vi "ManMarkZagueiro2.vi"(8 "Our Robot":T1={"id"=0, "function"=enum."Attacker", "x"=0.0, "y"=0.0, "orientation"=0.0, "v_tangent"=0.0, "v_normal"=0.0, "v_ang"=0.0, "kick_x"=0.0, "kick_z"=0.0, "dribble"=FALSE, "Timestamp"=timestamp(0 s since 1904-01-01), "estimatives"={"est_v_tangent"=0.0, "est_v_normal"=0.0, "est_vx"=0.0, "est_vy"=0.0, "Pos Robot Est"=[]}, "dest_x_kick"=0.0, "dest_y_kick"=0.0, "Gap Coord"=[], "States"=enum."GoToTangent", "Path "=[], "Path  Smooth"=[], "Dest"=[]}, 10 "IA Input":T6={"our_robots"=[], "enemy_robots"=[], "balls"=[], "geometry"={"line_width"=0, "field_length"=0, "field_width"=0, "boundary_width"=0, "referee_width"=0, "goal_width"=0, "goal_depth"=0, "goal_wall_width"=0, "center_circle_radius"=0, "defense_radius"=0, "defense_stretch"=0, "free_kick_from_defense_dist"=0, "penalty_spot_from_field_line_dist"=0, "penalty_line_from_spot_dist"=0}, "IA Judge"={"stage"="", "command"="", "our_goalie_id"=0.0, "enemy_goalie_id"=0.0, "command enum"=enum."Halt", "Time"=enum."Azul"}, "Received Timestamp"=timestamp(0 s since 1904-01-01), "Events"={"Touch"=FALSE, "Ball out"=FALSE, "id touch"=0.0, "Ball out of \nVision"=FALSE, "Ball inside \nGoalie area"=FALSE, "Robot not responding"=FALSE, "Robots responding status"=[1.0, 1.0, 1.0, 1.0, 1.0, 1.0], "Enemy Ball \nPossession"=FALSE, "Pass State"=FALSE, "id end of pass"=0.0, "Kick"=FALSE, "Id ini Possession"=0.0, "Ball Possesion"=FALSE, "Id Possesion"=0.0}}) -> (2 "Robot out":T1={"id"=0, "function"=enum."Attacker", "x"=0.0, "y"=0.0, "orientation"=0.0, "v_tangent"=0.0, "v_normal"=0.0, "v_ang"=0.0, "kick_x"=0.0, "kick_z"=0.0, "dribble"=FALSE, "Timestamp"=timestamp(0 s since 1904-01-01), "estimatives"={"est_v_tangent"=0.0, "est_v_normal"=0.0, "est_vx"=0.0, "est_vy"=0.0, "Pos Robot Est"=[]}, "dest_x_kick"=0.0, "dest_y_kick"=0.0, "Gap Coord"=[], "States"=enum."GoToTangent", "Path "=[], "Path  Smooth"=[], "Dest"=[]})   [LabVIEW 2017]
uses:
  Core/Field Size.ctl
  Core/AI Input.ctl
  Core/AI Robot.ctl
  Functions Enum.ctl
  AttackerStates.ctl
  Path Planning/RRT/PathDests.ctl
  Path Planning/RRT/PathDest.ctl
  Core/AI Ball.ctl
  Core/AI Judge.ctl
  Command Enum.ctl
  Util/Events/Events.ctl
panel:
  in  "Field Size in":T8
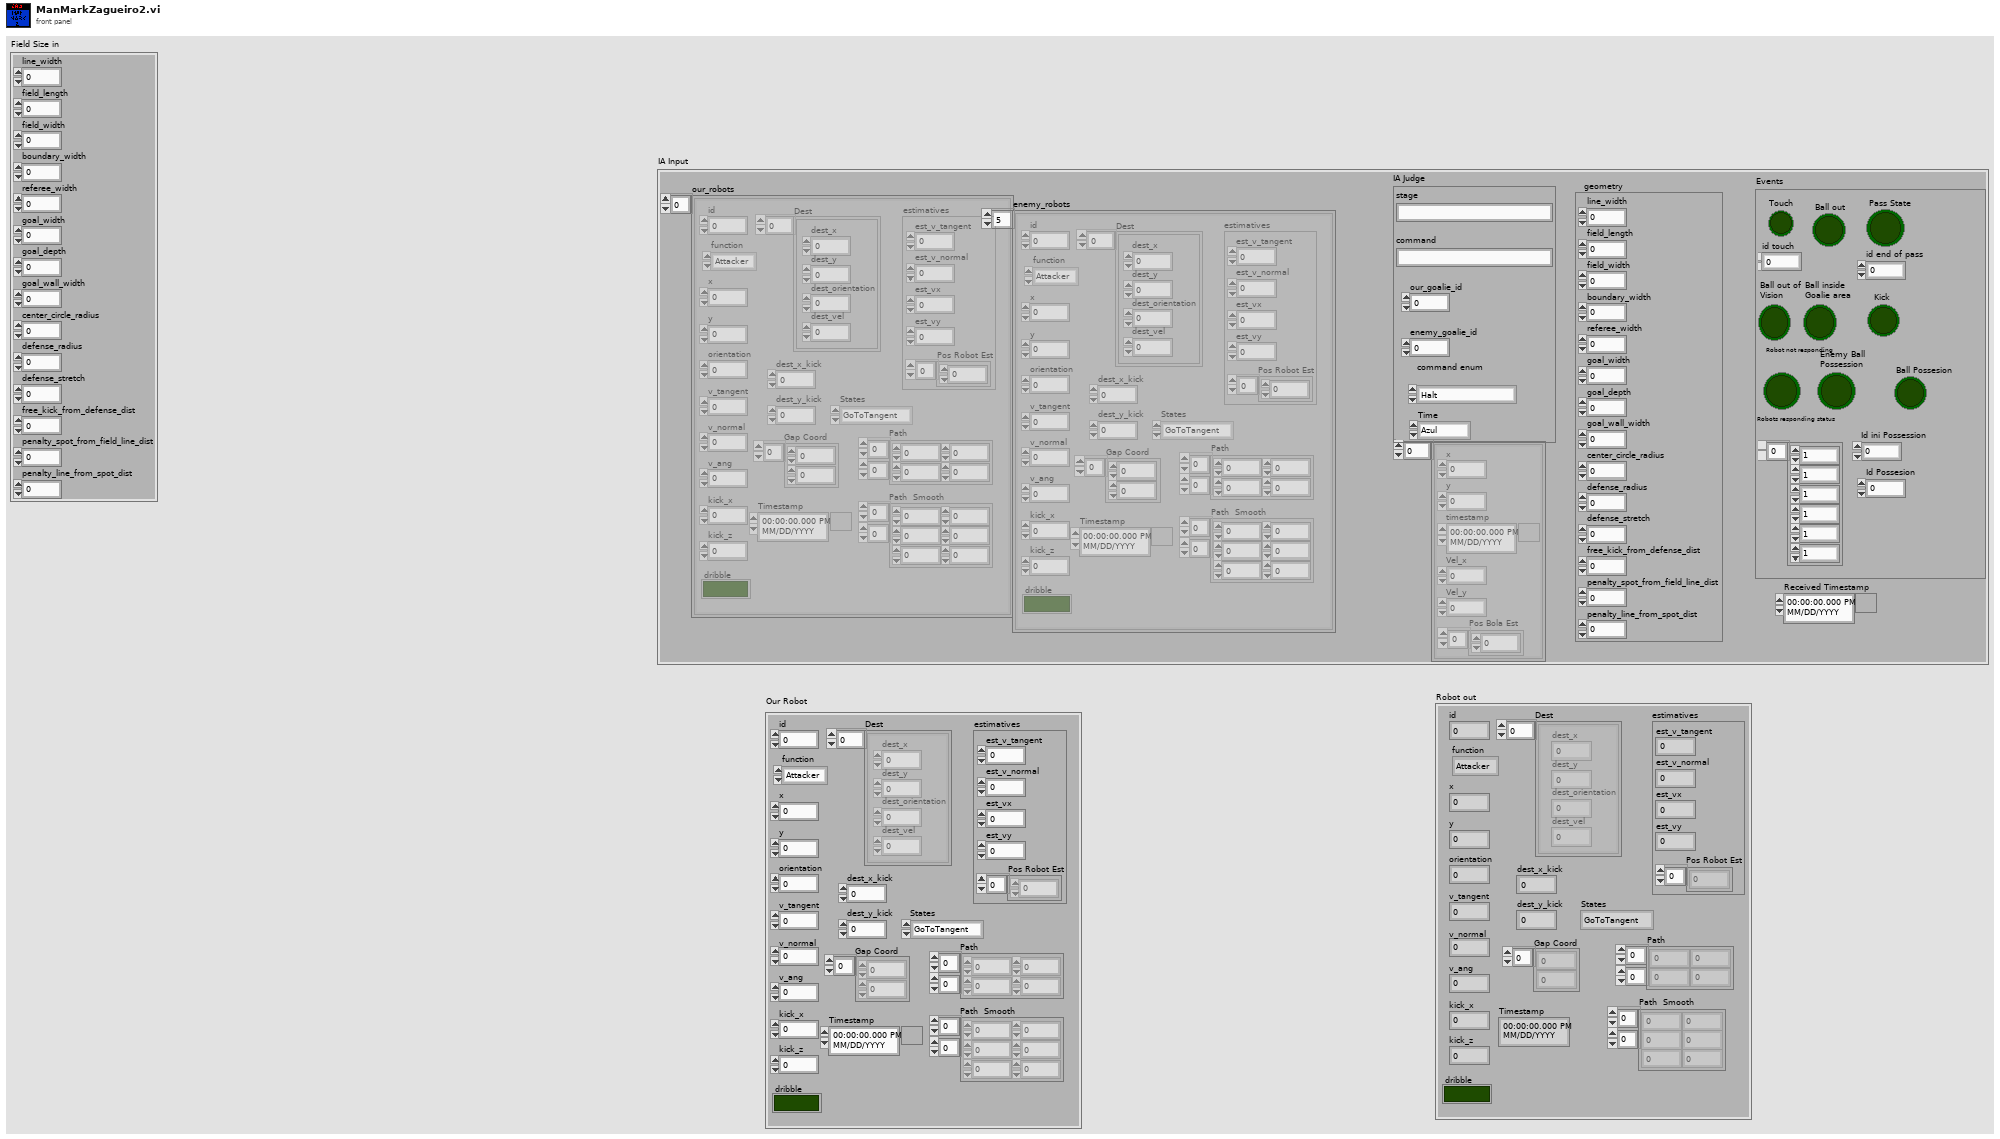
[diagram p1: front panel]
types:
  T1 = typedef "AI Robot.ctl" = cluster{"id":u32, "function":T2, "x":dbl, "y":dbl, "orientation":dbl, "v_tangent":dbl, "v_normal":dbl, "v_ang":dbl, "kick_x":dbl, "kick_z":dbl, "dribble":bool, "Timestamp":timestamp, "estimatives":cluster{"est_v_tangent":dbl, "est_v_normal":dbl, "est_vx":dbl, "est_vy":dbl, "Pos Robot Est":dbl[]}, "dest_x_kick":dbl, "dest_y_kick":dbl, "Gap Coord":dbl[], "States":T3, "Path ":dbl[][], "Path  Smooth":dbl[][], "Dest":T4}
  T2 = typedef "Functions Enum.ctl" = enum16{"Attacker", "Goalie", "Defender", "Striker", "Goto 0", "Dummy", "Kicker", "ZigZag"}
  T3 = typedef "AttackerStates.ctl" = enum16{"Pass", "GoToTangent", "BallGetting", "GoToKick", ""}
  T4 = typedef "PathDests.ctl" = T5[]
  T5 = typedef "PathDest.ctl" = cluster{"dest_x":dbl, "dest_y":dbl, "dest_orientation":dbl, "dest_vel":dbl}
  T6 = typedef "AI Input.ctl" = cluster{"our_robots":T1[], "enemy_robots":T1[], "balls":T7[], "geometry":T8, "IA Judge":T9, "Received Timestamp":timestamp, "Events":T11}
  T7 = typedef "AI Ball.ctl" = cluster{"x":dbl, "y":dbl, "timestamp":timestamp, "Vel_x":dbl, "Vel_y":dbl, "Pos Bola Est":dbl[]}
  T8 = typedef "Field Size.ctl" = cluster{"line_width":u32, "field_length":u32, "field_width":u32, "boundary_width":u32, "referee_width":u32, "goal_width":u32, "goal_depth":u32, "goal_wall_width":u32, "center_circle_radius":u32, "defense_radius":u32, "defense_stretch":u32, "free_kick_from_defense_dist":u32, "penalty_spot_from_field_line_dist":u32, "penalty_line_from_spot_dist":u32}
  T9 = typedef "AI Judge.ctl" = cluster{"stage":string, "command":string, "our_goalie_id":dbl, "enemy_goalie_id":dbl, "command enum":T10, "Time":enum16{"Azul", "Amarelo"}}
  T10 = typedef "Command Enum.ctl" = enum16{"Halt", "Stop", "Force Start", "PKA Normal Start", "Prepare Kickoff Ally", "PKE Normal Start", "Prepare Kickoff Enemy", "Prepare Penalty Ally", "PPA Normal Start", "Prepare Penalty Enemy", "PPE Normal Start", "Direct Free Enemy", "Direct Free Ally", "Indirect Free Enemy", "Indirect Free Ally", "Timeout Enemy", "Timeout Ally", "Goal Enemy", "Goal Ally", "Ball Placement Enemy", "Ball Placement Ally", "Normal Half Time", "Extra Time Break", "Extra Half Time", "None", "Post Game"}
  T11 = typedef "Events.ctl" = cluster{"Touch":bool, "Ball out":bool, "id touch":dbl, "Ball out of \nVision":bool, "Ball inside \nGoalie area":bool, "Robot not responding":bool, "Robots responding status":dbl[], "Enemy Ball \nPossession":bool, "Pass State":bool, "id end of pass":dbl, "Kick":bool, "Id ini Possession":dbl, "Ball Possesion":bool, "Id Possesion":dbl}
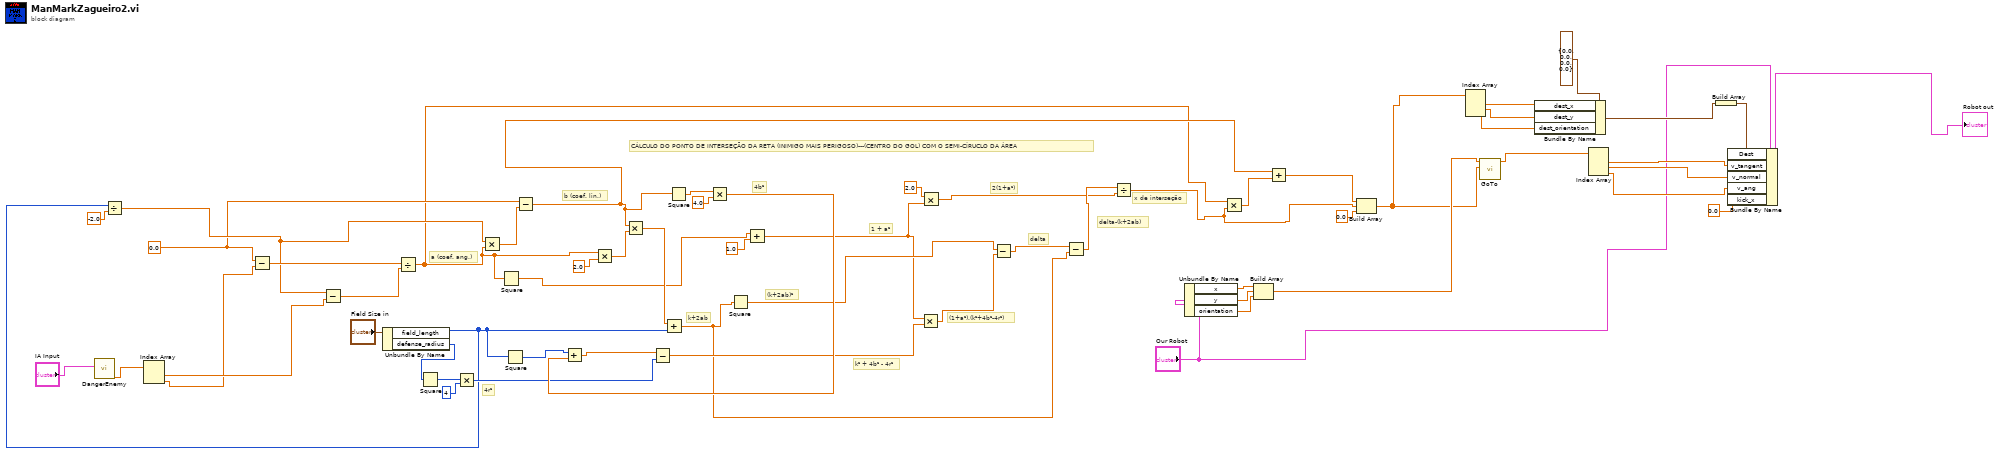
[diagram p0: block diagram]
diagram:
  w28 = 0.0
  # "x de interseção"
  # "CÁLCULO DO PONTO DE INTERSEÇÃO DA RETA (INIMIGO MAIS PERIGOSO)---(CENTRO DO GOL) COM O SEMI-CÍRUCLO DA ÁREA"
  # "delta-(k+2ab)"
  # "2(1+a²)"
  # "delta"
  # "(1+a²).(k²+4b²-4r²)"
  # "(k+2ab)²"
  # "k+2ab"
  # "k² + 4b² - 4r²"
  # "1 + a²"
  # "4r²"
  # "4b²"
  # "b (coef. lin.)"
  # "a (coef. ang.)"
  n1 = call "DangerEnemy.vi"("IA Input"="IA Input") -> ("Pos do segundo inimigo\nperigoso"=w3:dbl[])  [unwired: 7 in, 3 out]
  n2 = Index Array(array=w3) -> (element #1=w26:dbl, element #2=w25:dbl)  [unwired: 2 in]
  n3 = Subtract(x=w28, y=w25) -> (x-y=w59:dbl)
  n4 = Unbundle By Name("Field Size in") -> ("field_length"=w31:u32, "defense_radius"=w46:u32)
  n5 = Divide(x=w31, y=-2.0) -> (x/y=w29:dbl)
  n6 = Subtract(x=w29, y=w26) -> (x-y=w58:dbl)
  n7 = Divide(x=w59, y=w58) -> (x/y=w24:dbl)
  n8 = Square(x=w46) -> (x^2=w45:u32)
  n9 = Multiply(x=w45, y=u32 4) -> (x*y=w32:u32)
  n10 = Multiply(x=w29, y=w24) -> (x*y=w57:dbl)
  n11 = Square(x=w24) -> (x^2=w51:dbl)
  n12 = Square(x=w31) -> (x^2=w50:u32)
  n13 = Subtract(x=w28, y=w57) -> (x-y=w33:dbl)
  n14 = Multiply(x=w24, y=2.0 ("x")) -> (x*y=w54:dbl)
  n15 = Multiply(x=w33, y=w54) -> (x*y=w53:dbl)
  n16 = Add(x=w53, y=w31) -> (x+y=w38:dbl)
  n17 = Square(x=w33) -> (x^2=w49:dbl)
  n18 = Multiply(x=w49, y=4.0 ("x")) -> (x*y=w47:dbl)
  n19 = Add(x=w50, y=w47) -> (x+y=w43:dbl)
  n20 = Subtract(x=w43, y=w32) -> (x-y=w42:dbl)
  n21 = Square(x=w38) -> (x^2=w41:dbl)
  n22 = Add(x=w51, y=1.0) -> (x+y=w37:dbl)
  n23 = Multiply(x=w37, y=w42) -> (x*y=w40:dbl)
  n24 = Multiply(x=2.0 ("y"), y=w37) -> (x*y=w34:dbl)
  n25 = Subtract(x=w41, y=w40) -> (x-y=w39:dbl)
  n26 = Subtract(x=w39, y=w38) -> (x-y=w35:dbl)
  n27 = Divide(x=w35, y=w34) -> (x/y=w1:dbl)
  n28 = Unbundle By Name("Our Robot") -> ("x"=w20:dbl, "y"=w19:dbl, "orientation"=w18:dbl)
  n29 = Multiply(x=w24, y=w1) -> (x*y=w23:dbl)
  n30 = Build Array(w20, w19, w18) -> (w17:dbl[])
  n31 = Add(x=w33, y=w23) -> (x+y=w22:dbl)
  n32 = Build Array(w22, w1, 0.0 ("element")) -> (w15:dbl[])
  n33 = Index Array(array=w15) -> (element #1=w13:dbl, element #2=w12:dbl, element #3=w11:dbl)  [unwired: 3 in]
  n34 = call "GoTo.vi"("Target"=w15, "Position"=w17) -> ("Output\nVelocity"=w16:dbl[])  [unwired: 8 in, 1 out]
  n35 = Bundle By Name(cluster=T5 {"dest_x"=0.0, "dest_y"=0.0, "dest_orientation"=0.0, "dest_vel"=0.0} ("element"), "dest_x"=w13, "dest_y"=w12, "dest_orientation"=w11) -> (w9:T5)
  n36 = Index Array(array=w16) -> (element #1=w8:dbl, element #2=w7:dbl, element #3=w6:dbl)  [unwired: 3 in]
  n37 = Build Array(w9) -> (w10:T5[])
  n38 = Bundle By Name(cluster="Our Robot", "Dest"=w10, "v_tangent"=w8, "v_normal"=w7, "v_ang"=w6, "kick_x"=0.0) -> (→"Robot out":T1)
